vi "Modbus Connection Test.vi"(8 "error in (no error)":errorcluster caption="错误输入（无错误）", 10 "Protocol":enum16{"Serial Port", "Modbus TCP/IP"}(ring) caption="通讯方式", 11 "Modbus Info":T1={"Serial Port"="", "Baud Rate"=enum."19200", "Mode"=enum."RTU", "Parity"=0, "Unit ID"=1, "address"="", "port (502)"=502} {"Parity" items=["None", "Odd", "Even"]}) -> (0 "error out":errorcluster caption="错误输出")   [LabVIEW 2018]
uses:
  <vilib>/Modbus/master/Create Master Instance (Serial).vi
  <vilib>/Modbus/master/Create Master Instance (TCP).vi
  <vilib>/Modbus/master/Modbus Master.lvclass
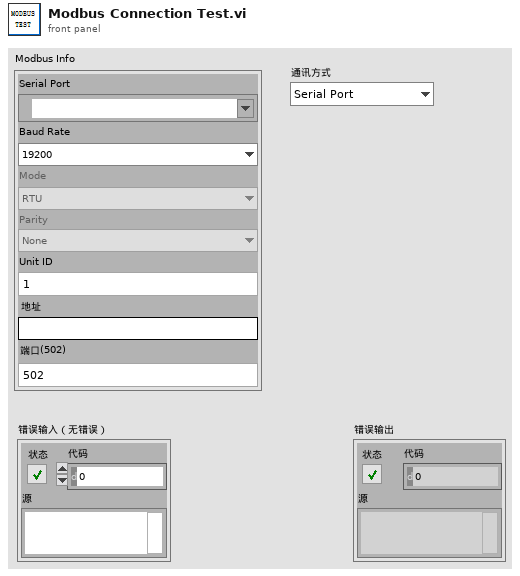
[diagram p1: front panel]
types:
  T1 = cluster{"Serial Port":refnum<visa-resource-name>, "Baud Rate":enum32{"1200", "2400", "4800", "9600", "19200", "38400", "57600", "115200"}, "Mode":enum16{"RTU", "ASCII"}, "Parity":u16, "Unit ID":u8, "address":string, "port (502)":u16}
  T2 = enum32{"1200", "2400", "4800", "9600", "19200", "38400", "57600", "115200"}
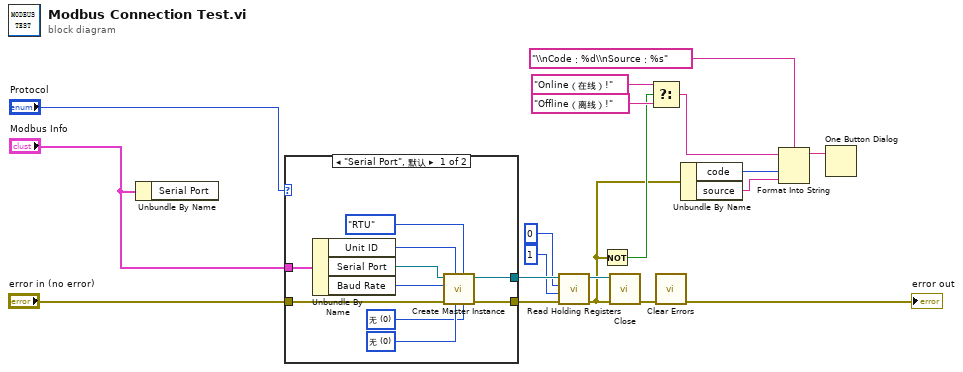
[diagram p0: block diagram]
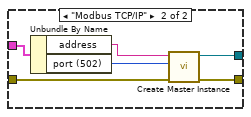
[diagram p2: hidden frame]
diagram:
  n1 = Unbundle By Name("Modbus Info") -> ()  [unwired: 1 out]
  n2 = case shown="\"Serial Port\", 默认" "Protocol" {
    tunnel: [w25 w35] -> w16
    tunnel: [w26 w34] -> w15
    tunnel: "error in (no error)" -> [w24 w33]
    tunnel: "Modbus Info" -> [w20 w31]
    frame "Serial Port", Default {
      w27 = u16 0 items=["无", "XON/XOFF", "RTS/CTS", "XON/XOFF & RTS/CTS", "DTR/DSR", "XON/XOFF & DTR/DSR"] ("flow control (None)")
      w28 = u16 0 items=["无", "奇", "偶"] ("parity (Even)")
      n3 = Unbundle By Name(w20) -> ("Unit ID"=w21:u8, "Serial Port"=w23:refnum<visa-resource-name>, "Baud Rate"=w22:T2)
      n4 = call-poly <vilib>:"Create Master Instance.vi"("flow control (None)"=w27, "serial type"=enum16{"RTU", "ASCII"}."RTU", "parity (Even)"=w28, "unit ID"=w21, "error in (no error)"=w24, "baud rate (9600)"=w22, "VISA resource name"=w23) -> ("error out"=w26:errorcluster, "serial master instance"=w25:refnum<class "Modbus Master.lvclass">)  [unwired: 3 in]
    }
    frame "Modbus TCP/IP" {
      n5 = Unbundle By Name(w31) -> ("address"=w30:string, "port (502)"=w32:u16)
      n6 = call-poly <vilib>:"Create Master Instance.vi"("error in (no error)"=w33, "port (502)"=w32, "address"=w30) -> ("error out"=w34:errorcluster, "TCP master instance"=w35:refnum<class "Modbus Master.lvclass">)  [unwired: 7 in]
    }
  }
  n7 = call-dynamic "Read Holding Registers.vi"("error in (no error)"=w15, "number of holding registers"=u16 1, "starting address"=u16 0, "Modbus master in"=w16) -> ("error out"=w8:errorcluster, "Modbus master out"=w12:refnum<class "Modbus Master.lvclass">)  [unwired: 5 in, 1 out]
  n8 = Not(x=w8) -> (.not. x?=w17:bool)
  n9 = call-dynamic "Close.vi"("error in (no error)"=w8, "Modbus master in"=w12) -> ("error out"=w9:errorcluster)  [unwired: 9 in]
  n10 = Select(t="Online（在线）!", s=w17, f="Offline（离线）!") -> (s? t:f=w5:string)
  n11 = call <vilib>:"Clear Errors.vi"("error in (no error)"=w9) -> ("error out"=→"error out":errorcluster)  [unwired: 5 in, 1 out]
  n12 = Unbundle By Name(w8) -> ("code"=w7:i32, "source"=w6:string)
  n13 = Format Into String(format string="\\nCode：%d\\nSource：%s" ("格式字符串"), initial string=w5, w7, w6) -> (resulting string=w4:string)  [unwired: 1 in, 1 out]
  n14 = One Button Dialog(message=w4) -> ()  [unwired: 1 in, 1 out]
